vi "rad_Deploy Application Image.vi"(7 "App Image Temp Folder":path=path "C:/dev/Architectures/Reference Designs/Application Deployment and Replication/Application Deployment Utility/trunk/source/Application Images/_temp", 8 "error in (no error)":errorcluster, 10 "Selected Targets":T1[](array[typedef]) {"Primary NIC"."IP Address Request Mode" items=["Static"=1, "DHCP/Link-Local"=2, "Link-Local Only"=4, "DHCP Only"=8]}, 11 "App Image Path":path=path "C:/dev/Architectures/Reference Designs/Application Deployment and Replication/Application Deployment Utility/trunk/source/Application Images/AppImage1.lvappimg") -> (0 "error out":errorcluster, 1 "Cancelled":bool)   [LabVIEW 2020]
uses:
  TypeDefs/rad_Target Configuration Operations.ctl
  TypeDefs/rad_Deployment Status Data Type.ctl
  Util/FP Control/FP Control Functions.ctl
  TypeDefs/rad_Deployment Progress Data Type.ctl
  TypeDefs/rad_Deployment Notifiers.ctl
  <vilib>/nisyscfg/nisyscfg.lvlib
  <vilib>/nisyscfg/Close (System).vi
  support/SubVIs/Target Information.ctl
  Targets/TypeDefs/rad_Target Network Settings.ctl
  TypeDefs/rad_Target Configuration Settings.ctl
panel:
  in  "Configure Targets":bool
  out "Stop Updates":bool
  in  "Deploy":bool
  in  "Log":bool
  in  "Stop":bool
  in  "State Variables":T6={"App Image Path"=path "C:/dev/Architectures/Reference Designs/Application Deployment and Replication/Application Deployment Utility/trunk/source/Application Images/AppImage1.lvappimg", "App Image Temp Folder"=path "C:/dev/Architectures/Reference Designs/Application Deployment and Replication/Application Deployment Utility/trunk/source/Application Images/_temp", "Targets"=[], "Target Configuration Options"={"NumInBatch"=0, "Target Config Operation"=enum."No Config", "Target Name"="", "Increment Static IPs"=FALSE, "Change Target Name"=FALSE, "Primary NIC"={"MAC address"="", "IP Address Request Mode"=2, "IP address"="", "Subnet mask"="", "Gateway"="", "DNS server"=""}}, "Deployment Notifiers"=[]} {"Target Configuration Options"."Primary NIC"."IP Address Request Mode" items=["Static"=1, "DHCP/Link-Local"=2, "Link-Local Only"=4, "DHCP Only"=8]; "Targets"."Primary NIC"."IP Address Request Mode" items=["Static"=1, "DHCP/Link-Local"=2, "Link-Local Only"=4, "DHCP Only"=8]}
  out "Targets":i32(listbox)
  in  "Close":bool
  # "Targets"
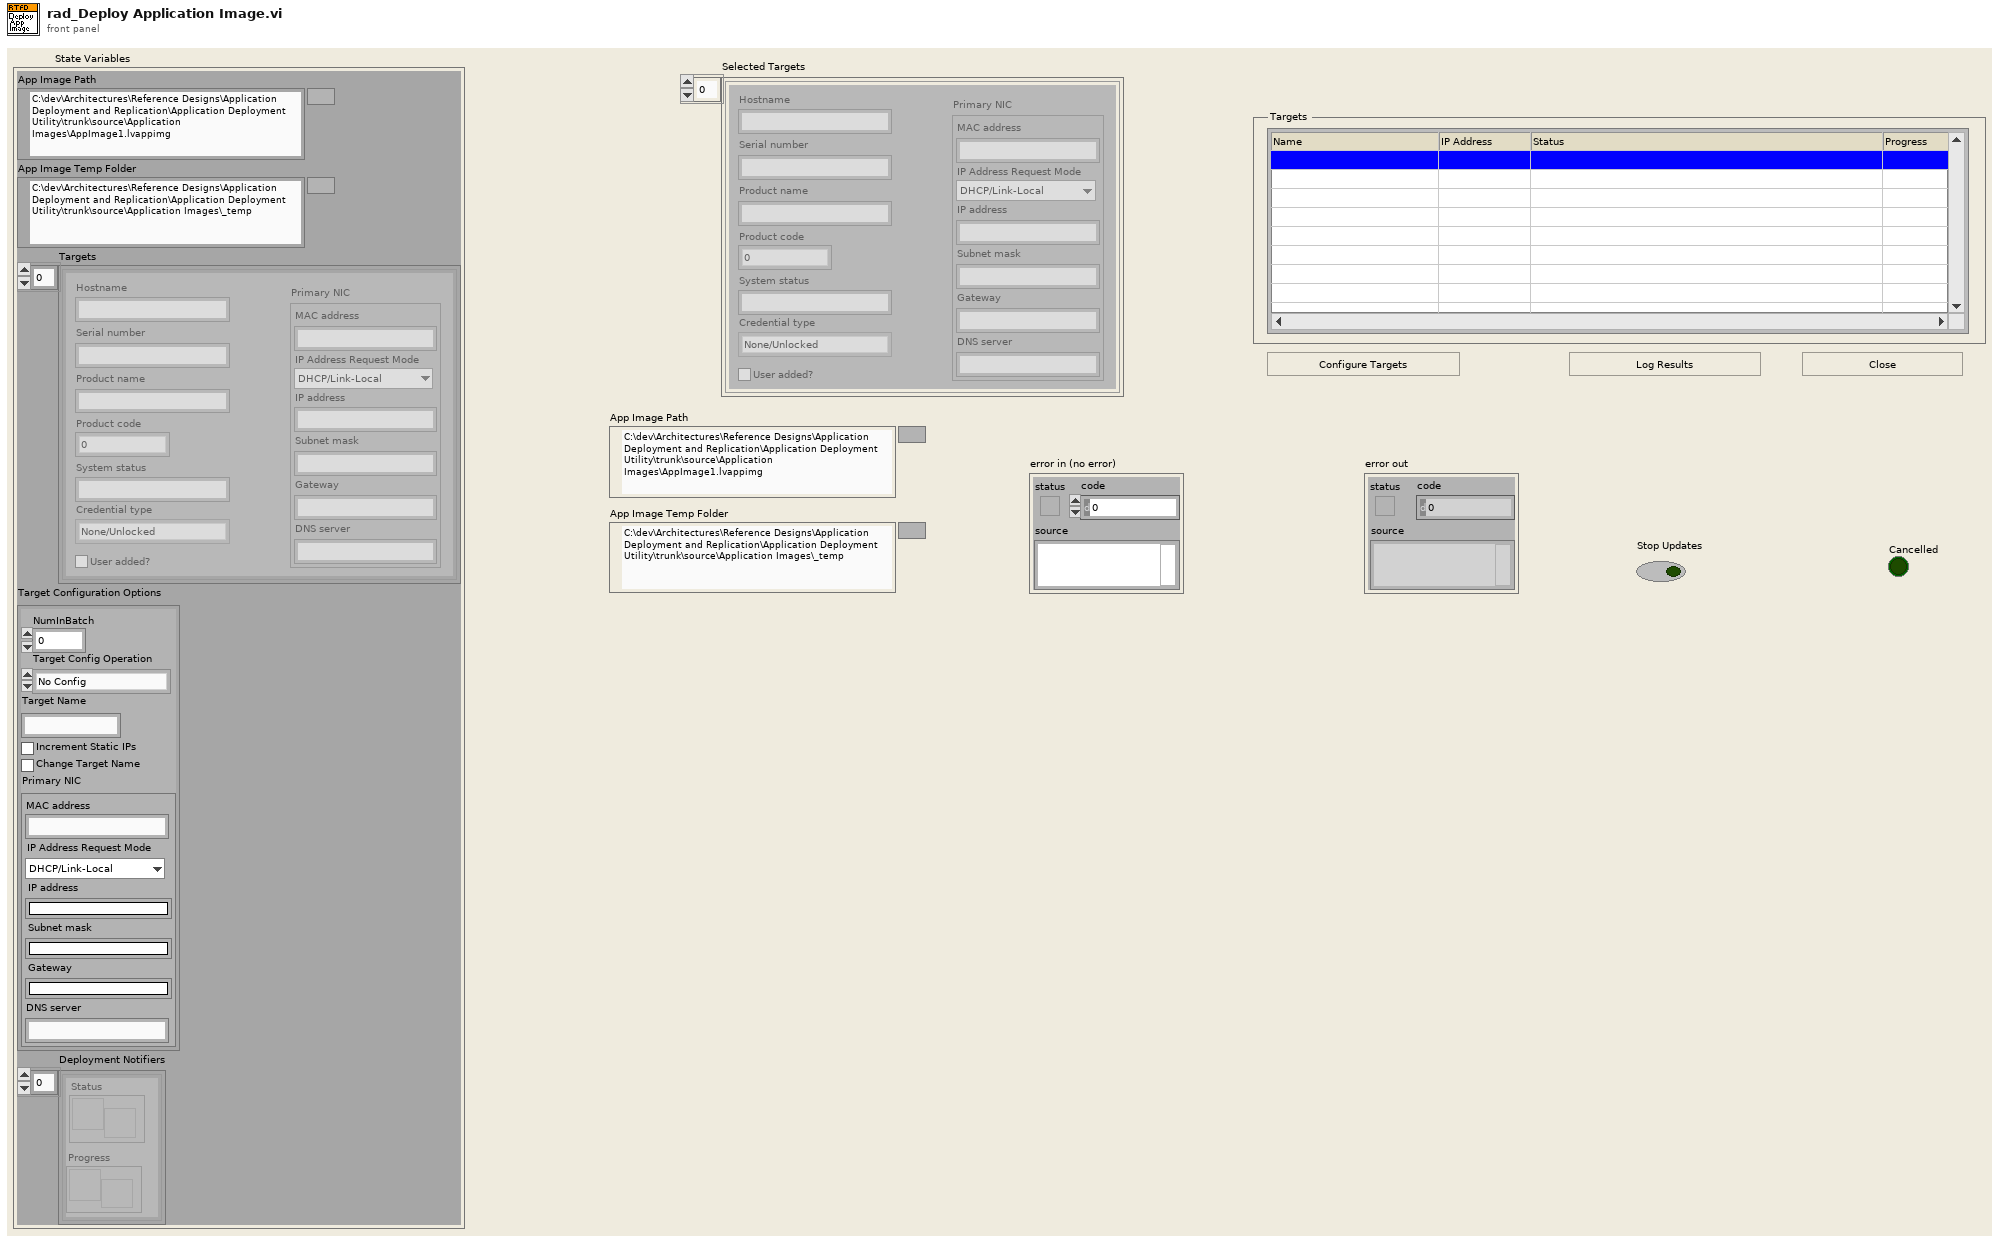
[diagram p1: front panel]
types:
  T1 = typedef "Target Information.ctl" = cluster{"Hostname":string, "Serial number":string, "Product name":string, "Product code":i32, "System status":string, "Credential type":enum16{"None/Unlocked", "FTP Password", "NIAuth Credentials"}, "User added?":bool, "Primary NIC":T2}
  T2 = typedef "rad_Target Network Settings.ctl" = cluster{"MAC address":string, "IP Address Request Mode":i32, "IP address":string, "Subnet mask":string, "Gateway":string, "DNS server":string}
  T3 = typedef "rad_Target Configuration Settings.ctl" = cluster{"NumInBatch":u32, "Target Config Operation":T4, "Target Name":string, "Increment Static IPs":bool, "Change Target Name":bool, "Primary NIC":T2}
  T4 = typedef "rad_Target Configuration Operations.ctl" = enum8{"No Config", "Image Config", "Static Config"}
  T5 = typedef "rad_Deployment Notifiers.ctl" = cluster{"Status":refnum<notifier>, "Progress":refnum<notifier>}
  T6 = cluster{"App Image Path":path, "App Image Temp Folder":path, "Targets":T1[], "Target Configuration Options":T3, "Deployment Notifiers":T5[]}
  T7 = typedef "rad_Deployment Progress Data Type.ctl" = i8
  T8 = typedef "rad_Deployment Status Data Type.ctl" = string
  T9 = typedef "FP Control Functions.ctl" = enum16{"Open", "Close", "Bring To Front", "Center"}
  T10 = enum8{"Enabled", "Disabled", "Disabled and Grayed Out"}
  T11 = typedef "rad_Application Image Properties.ctl" = cluster{"Name":string, "Version":string, "Time":timestamp, "Description":string, "Key":string, "Chassis":string, "FPGA Properties":T12, "Model":string, "Retrieve":string[], "Deploy":string[], "Installed Software":string[]}
  T12 = typedef "rad_FPGA Properties.ctl" = T13[]
  T13 = typedef "rad_FPGA Flash Properties.ctl" = cluster{"Resource Name":string, "Path":path}
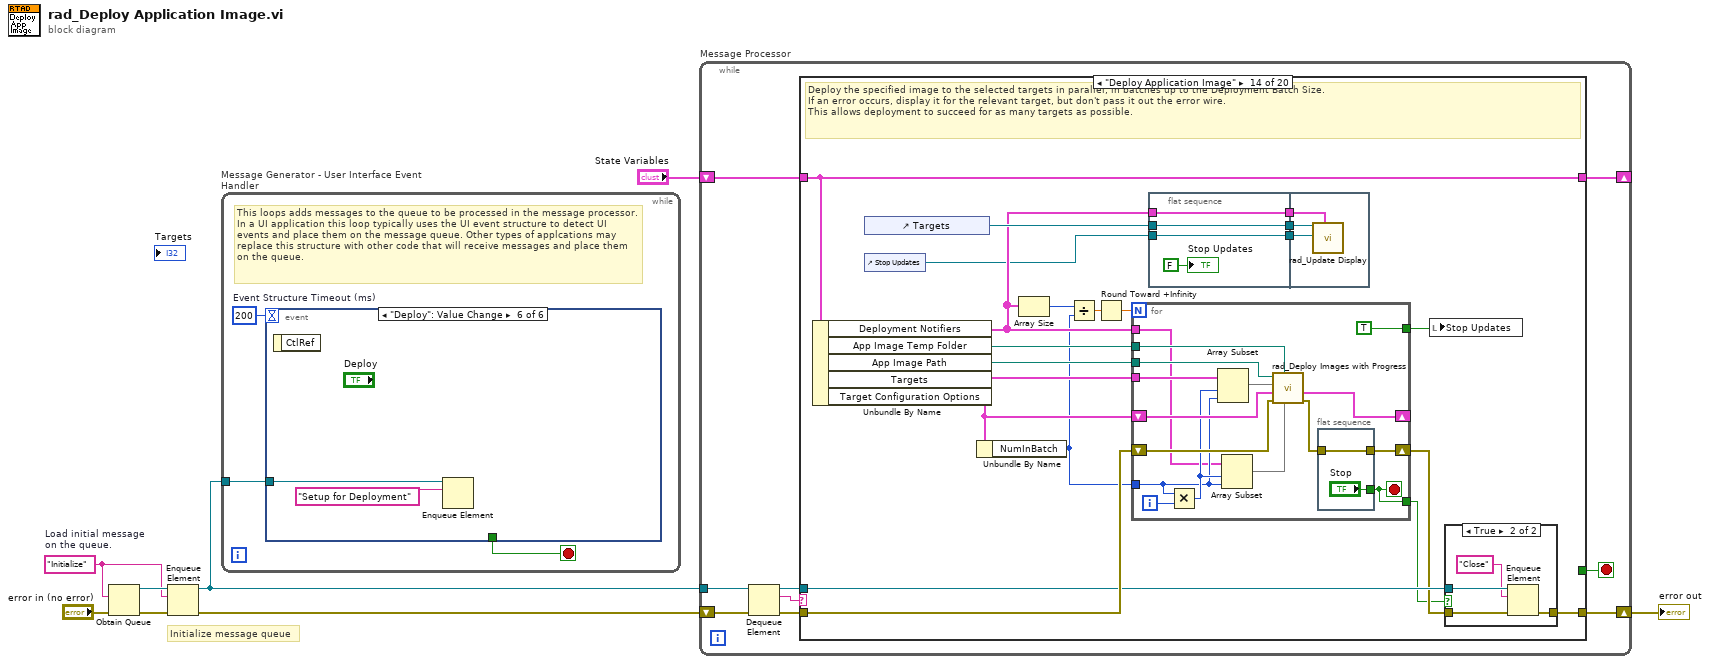
[diagram p0: block diagram]
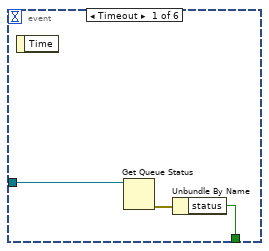
[diagram p2: hidden frame]
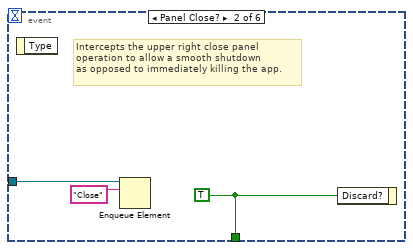
[diagram p3: hidden frame]
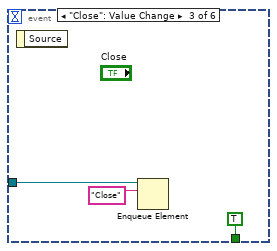
[diagram p4: hidden frame]
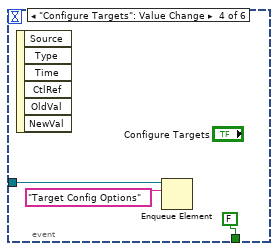
[diagram p5: hidden frame]
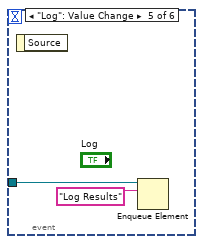
[diagram p6: hidden frame]
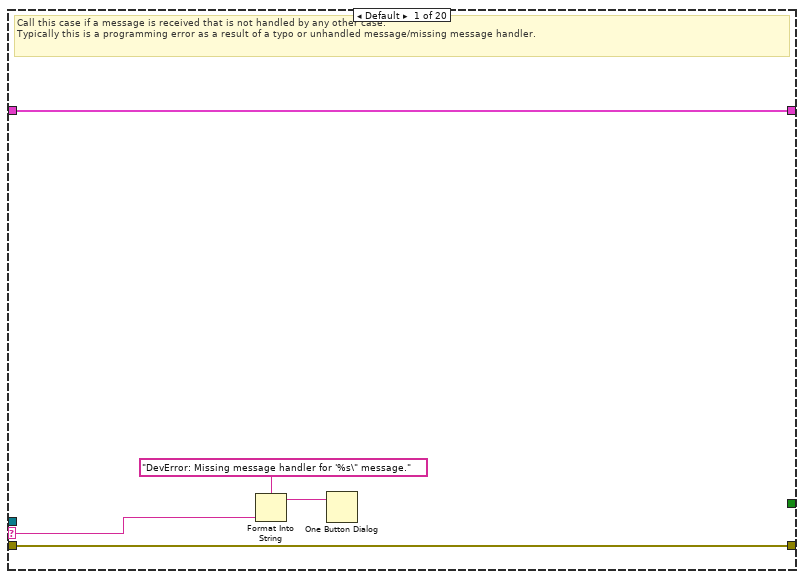
[diagram p7: hidden frame]
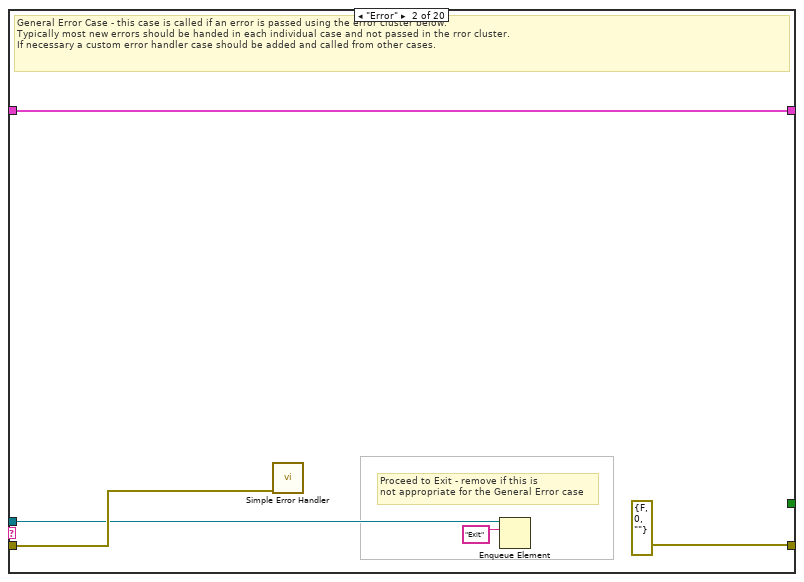
[diagram p8: hidden frame]
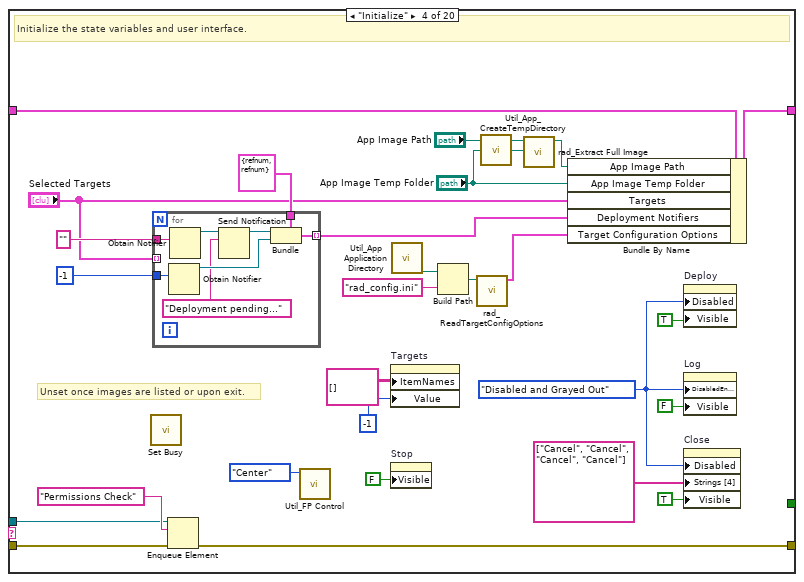
[diagram p10: hidden frame]
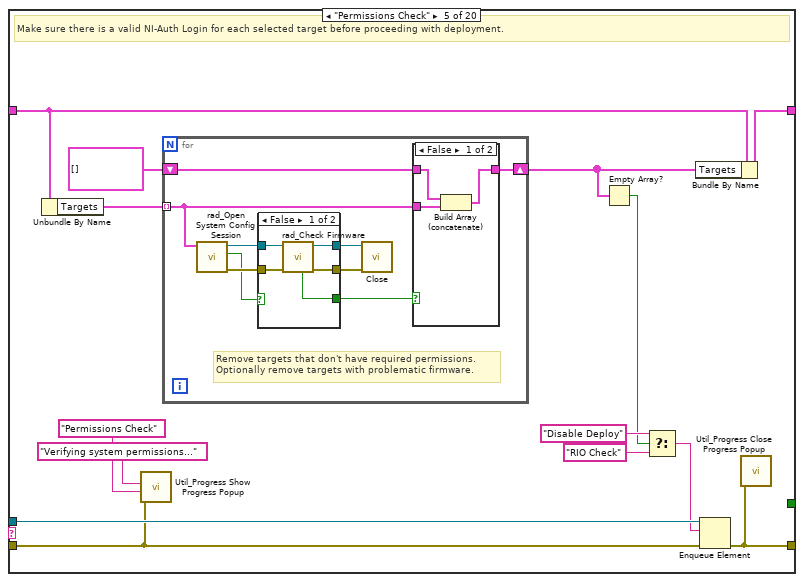
[diagram p11: hidden frame]
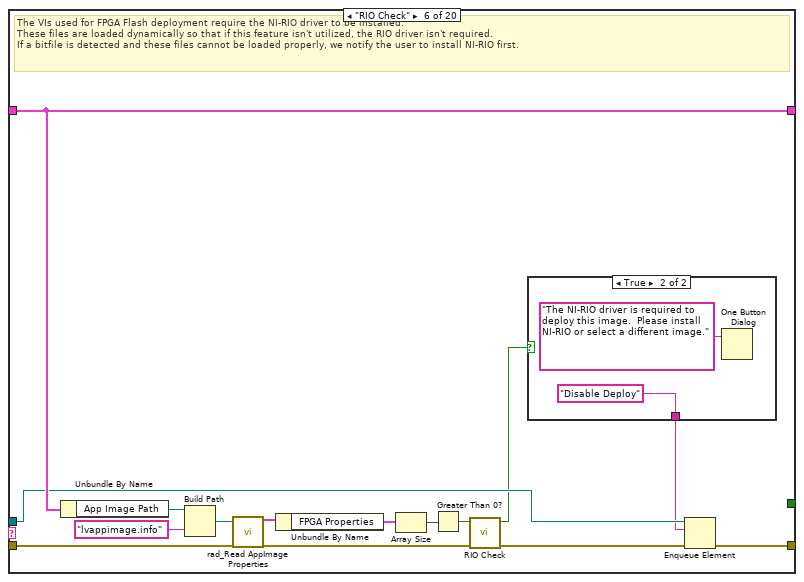
[diagram p14: hidden frame]
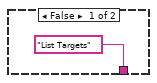
[diagram p15: hidden frame]
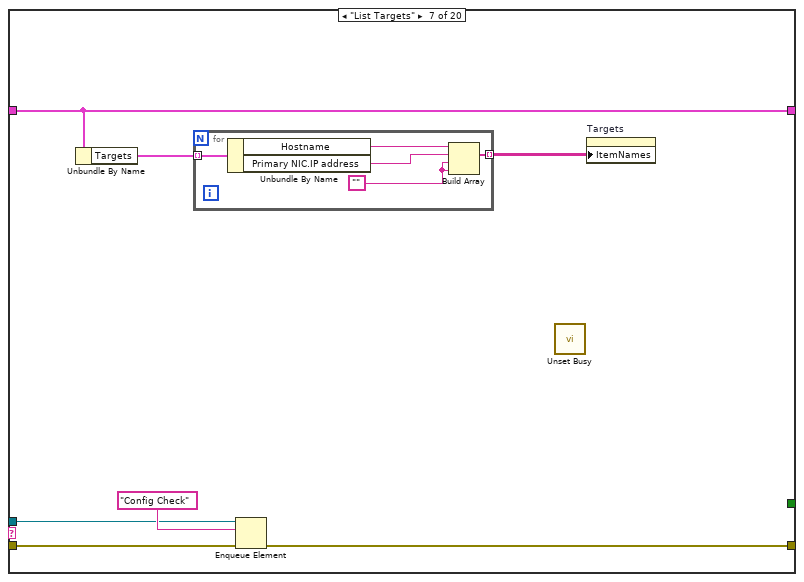
[diagram p16: hidden frame]
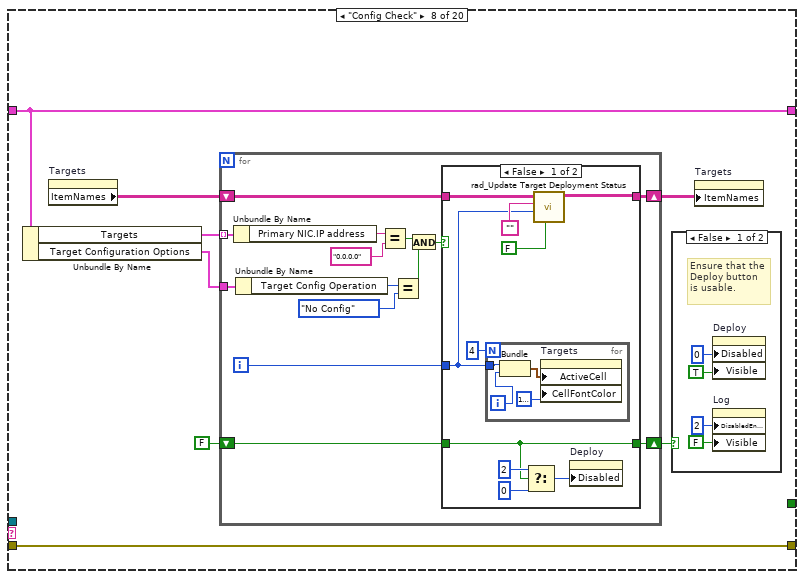
[diagram p17: hidden frame]
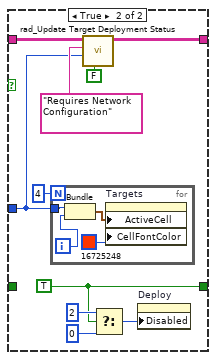
[diagram p19: hidden frame]
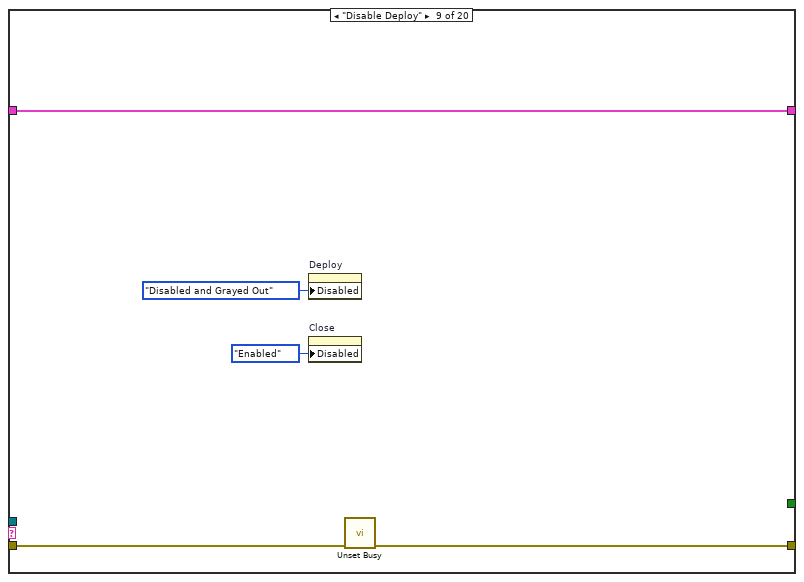
[diagram p20: hidden frame]
diagram:
  w1 = "Initialize"  # Load initial message on the queue.
  # "Initialize message queue"
  n1 = Obtain Queue(element data type=w1, error in (no error)="error in (no error)") -> (queue out=w3:refnum<queue>, error out=w8:errorcluster)  [unwired: 3 in, 1 out]
  n2 = Enqueue Element(queue=w3, element=w1, error in (no error)=w8) -> (queue out=w2:refnum<queue>, error out=w4:errorcluster)  [unwired: 1 in, 1 out]
  n3 = while "Message Generator - User Interface Event Handler" {
    tunnel: w2 -> [w9]
    stop <- w10 stop-if-true
    w11 = 200  # Event Structure Timeout (ms)
    # "This loops adds messages to the queue to be processed in the message processor. In a UI application this loop typically uses the UI event structure to detect UI events and place them on the message queue. Other types of applcations may replace this structure with other code that will receive messages and place them on the queue."
    n4 = event shown="[5] \"Deploy\": Value Change" {
      selector: _ -> [_ _ _ _ _ _]
      dyn-events: _ -> [_ _ _ _ _ _]
      timeout: w11 -> [_ _ _ _ _ _]
      tunnel: [w13 w17 TRUE ("Discard?") FALSE ("Discard?") _ _] -> w10
      tunnel: w9 -> [w12 w16 w20 w23 w25 w27]
      event Timeout {
        n5 = event-data() -> ()  [unwired: 2 out]
        n6 = Get Queue Status(queue=w12) -> (error out=w14:errorcluster)  [unwired: 2 in, 7 out]
        n7 = Unbundle By Name(w14) -> ("status"=w13:bool)
      }
      event Panel Close? {
        w17 = TRUE ("Discard?")
        # "Intercepts the upper right close panel\noperation to allow a smooth shutdown\nas opposed to immediately killing the app."
        n8 = event-data() -> ()  [unwired: 2 out]
        n9 = Enqueue Element(queue=w16, element="Close") -> ()  [unwired: 2 in, 3 out]
        n10 = event-data("Discard?"=w17) -> ()  [unwired: 1 in, 1 out]
      }
      event "Close": Value Change {
        n11 = event-data() -> ()  [unwired: 2 out]
        n12 = Enqueue Element(queue=w20, element="Close") -> ()  [unwired: 2 in, 3 out]
      }
      event "Configure Targets": Value Change {
        n13 = event-data() -> ()  [unwired: 7 out]
        n14 = Enqueue Element(queue=w23, element="Target Config Options") -> ()  [unwired: 2 in, 3 out]
      }
      event "Log": Value Change {
        n15 = event-data() -> ()  [unwired: 2 out]
        n16 = Enqueue Element(queue=w25, element="Log Results") -> ()  [unwired: 2 in, 3 out]
      }
      event "Deploy": Value Change {
        n17 = event-data() -> ()  [unwired: 2 out]
        n18 = Enqueue Element(queue=w27, element="Setup for Deployment") -> ()  [unwired: 2 in, 3 out]
      }
    }
  }
  n19 = while "Message Processor" {
    shift-left: w4 -> [w31]
    shift-right: [w32] -> w5
    tunnel: w2 -> [w30]
    shift-left: "State Variables" -> [w36]
    shift-right: [w35] -> _
    stop <- w28 stop-if-true
    n20 = Dequeue Element(queue=w30, error in (no error)=w31) -> (queue out=w34:refnum<queue>, element=w29:string, error out=w33:errorcluster)  [unwired: 1 in, 1 out]
    n21 = case shown="\"Deploy Application Image\"" w29 {
      selector: w29 -> [w39 _ _ _ _ _ _ _ _ _ _ _ _ _ _ _ _ _ _ _]
      tunnel: [w41 w46 w48 w75 w95 w131 w142 w152 w206 w210 w212 w218 w238 w257 w294 w302 w304 w312 w315 w322] -> w35
      tunnel: w36 -> [w41 w46 w48 w76 w96 w131 w142 w152 w206 w210 w212 w219 w238 w257 w294 w302 w304 w312 w315 w322]
      tunnel: w34 -> [_ w43 _ w54 w94 w128 w138 _ _ _ _ w216 w234 w252 _ _ _ w306 _ w327]
      tunnel: w33 -> [w40 w44 w47 w70 w90 w123 w140 w157 w208 w209 w211 w220 w239 w256 w295 w300 w303 w307 w313 w328]
      tunnel: [w40 errorcluster {"status"=FALSE, "code"=0, "source"=""} ("error out") w47 w56 w89 w129 w139 w157 w207 w209 w211 w214 w230 w250 w295 w299 w303 w305 w313 w319] -> w32
      tunnel: [_ _ _ _ _ _ _ _ _ _ _ _ _ _ _ _ _ _ _ TRUE] -> w28
      frame Default {
        # "Call this case if a message is received that is not handled by any other case.\nTypically this is a programming error as a result of a typo or unhandled message/missing message handler."
        n22 = Format Into String(format string="DevError: Missing message handler for '%s\" message." ("message"), w39) -> (resulting string=w37:string)  [unwired: 2 in, 1 out]
        n23 = One Button Dialog(message=w37) -> ()  [unwired: 2 out]
      }
      frame "Error" {
        # "Proceed to Exit - remove if this is\nnot appropriate for the General Error case"
        # "General Error Case - this case is called if an error is passed using the error cluster below.\nTypically most new errors should be handed in each individual case and not passed in the rror cluster.\nIf necessary a custom error handler case should be added and called from other cases."
        n24 = call <vilib>:"Simple Error Handler.vi"("error in (no error)"=w44) -> ()  [unwired: 1 in, 8 out]
        n25 = Enqueue Element(queue=w43, element="Exit") -> ()  [unwired: 2 in, 3 out]
      }
      frame "*******Init******" {
        # "Dummy case to add a seperator in the Case Structure menu."
      }
      frame "Initialize" {
        w49 = T10."Disabled and Grayed Out" ("Disabled")
        # "Unset once images are listed or upon exit."
        # "Initialize the state variables and user interface."
        n26 = call <vilib>:"Set Busy.vi"() -> ()  [unwired: 10 in, 2 out]
        n27 = for {
          tunnel: T8 "" ("status notifier data type") -> [w84]
          tunnel: T7 -1 ("Progress") -> [w83]
          tunnel: T5 {"Status"=refnum, "Progress"=refnum} ("Deployment Notifiers") -> [w81]
          tunnel: [w80] -> w65 mode=indexing
          tunnel: "Selected Targets" -> [_] mode=indexing
          n28 = Obtain Notifier(notification data type=w83) -> (notifier out=w82:refnum<notifier>)  [unwired: 3 in, 2 out]
          n29 = Obtain Notifier(notification data type=w84) -> (notifier out=w79:refnum<notifier>)  [unwired: 3 in, 2 out]
          n30 = Send Notification(notification=T8 "Deployment pending...", notifier=w79) -> (notifier out=w78:refnum<notifier>)  [unwired: 1 in, 1 out]
          n31 = Bundle(cluster=w81, "Status"=w78, "Progress"=w82) -> (w80:T5)
        }
        n32 = Enqueue Element(queue=w54, element="Permissions Check", error in (no error)=w70) -> (error out=w56:errorcluster)  [unwired: 1 in, 2 out]
        n33 = call "Util_FP Control.vi"("Function"=FP_Control_Functions."Center") -> ()  [unwired: 1 in, 10 out]
        n34 = property on="Targets" class="MCListbox (strict)"("ItemNames"=string[][] [] ("Item Names"), "Value"=-1 ("Targets")) -> ()  [unwired: 2 in, 2 out]
        n35 = property on="Stop" class="Bool"("Visible"=FALSE) -> ()  [unwired: 2 in, 2 out]
        n36 = call "Util_App Application Directory.vi"() -> ("Application Directory"=w64:path)  [unwired: 11 out]
        n37 = Build Path(base path=w64, name or relative path="rad_config.ini" ("Config File Name")) -> (appended path=w62:path)
        n38 = call "rad_ReadTargetConfigOptions.vi"("configuration file path"=w62) -> ("TargetConfigurationOptions"=w61:T3)  [unwired: 9 in, 1 out]
        n39 = call "Util_App_CreateTempDirectory.vi"("TempFolderPath"="App Image Temp Folder") -> ("TempFolderPath_out"=w58:path)
        n40 = call "rad_Extract Full Image.vi"("App Image Temp Folder"=w58, "Zipped App Image File Path"="App Image Path") -> ("Unzipped App Image Folder Path"=w59:path)  [unwired: 8 in, 1 out]
        n41 = Bundle By Name(cluster=w76, "App Image Path"=w59, "App Image Temp Folder"="App Image Temp Folder", "Targets"="Selected Targets", "Deployment Notifiers"=w65, "Target Configuration Options"=w61) -> (w75:T6)
        n42 = property on="Deploy" class="Bool"("Disabled"=w49, "Visible"=TRUE) -> ()  [unwired: 2 in, 2 out]
        n43 = property on="Log" class="Bool"("DisabledEnum"=w49, "Visible"=FALSE) -> ()  [unwired: 2 in, 2 out]
        n44 = property on="Close" class="Bool"("Disabled"=w49, "Strings [4]"=string[] ["Cancel", "Cancel", "Cancel", "Cancel"], "Visible"=TRUE) -> ()  [unwired: 2 in, 2 out]
      }
      frame "Permissions Check" {
        # "Make sure there is a valid NI-Auth Login for each selected target before proceeding with deployment."
        n45 = Unbundle By Name(w96) -> ("Targets"=w98:T1[])
        n46 = call "Util_Progress Show Progress Popup.vi"("error in (no error)"=w90, "Title"="Permissions Check" ("Message"), "Message"="Verifying system permissions...") -> ()  [unwired: 8 in, 1 out]
        n47 = for {
          tunnel: w98 -> [w105] mode=indexing
          shift-right: [w107] -> w86
          shift-left: T1[] [] -> [w106]
          # "Remove targets that don't have required permissions.\nOptionally remove targets with problematic firmware."
          n48 = call "rad_Open System Config Session.vi"("Target settings"=w105) -> ("error out"=w104:errorcluster, "Cancelled"=w99:bool, "Session out"=w102:refnum<k21>)  [unwired: 7 in, 1 out]
          n49 = case shown="False" w99 {
            selector: w99 -> [_ w113]
            tunnel: w104 -> [w112 w115]
            tunnel: [w109 w115] -> w103
            tunnel: w102 -> [w111 w114]
            tunnel: [w110 w114] -> w101
            tunnel: [w108 w113] -> w100
            frame False {
              n50 = call "rad_Check Firmware.vi"("error in (no error)"=w112, "System Configuration"=w111) -> ("error out"=w109:errorcluster, "System Configuration out"=w110:refnum<k21>, "Bad firmware and user canceled"=w108:bool)  [unwired: 7 in]
            }
            frame True {
            }
          }
          n51 = call-poly <vilib>:"Close.vi"("error in (no error)"=w103, "Session in"=w101) -> ()  [unwired: 9 in, 1 out]
          n52 = case shown="False" w100 {
            tunnel: w105 -> [w118 _]
            tunnel: [w117 w119] -> w107
            tunnel: w106 -> [w116 w119]
            frame False {
              n53 = Build Array (concatenate)(w116, w118) -> (w117:T1[])
            }
            frame True {
            }
          }
        }
        n54 = Empty Array?(array=w86) -> (empty?=w85:bool)
        n55 = Select(t="Disable Deploy", s=w85, f="RIO Check") -> (s? t:f=w91:string)
        n56 = Bundle By Name(cluster=w96, "Targets"=w86) -> (w95:T6)
        n57 = Enqueue Element(queue=w94, element=w91, error in (no error)=w90) -> (error out=w89:errorcluster)  [unwired: 1 in, 2 out]
        n58 = call "Util_Progress Close Progress Popup.vi"("error in (no error)"=w89) -> ()  [unwired: 10 in, 1 out]
      }
      frame "RIO Check" {
        # "The VIs used for FPGA Flash deployment require the NI-RIO driver to be installed.  \nThese files are loaded dynamically so that if this feature isn't utilized, the RIO driver isn't required.\nIf a bitfile is detected and these files cannot be loaded properly, we notify the user to install NI-RIO first."
        n59 = Unbundle By Name(w131) -> ("App Image Path"=w121:path)
        n60 = Build Path(base path=w121, name or relative path="lvappimage.info") -> (appended path=w120:path)
        n61 = call "rad_Read AppImage Properties.vi"("AppImage Properties Path"=w120, "error in (no error)"=w123) -> ("AppImage Properties"=w124:T11, "error out"=w125:errorcluster)  [unwired: 12 in, 4 out]
        n62 = Unbundle By Name(w124) -> ("FPGA Properties"=w134:T12)
        n63 = Array Size(array=w134) -> (size(s)=w133:i32)
        n64 = Greater Than 0?(x=w133) -> (x > 0?=w132:bool)
        n65 = call "RIO Check.vi"("error in"=w125, "Requires RIO"=w132) -> ("error out"=w130:errorcluster, "RIO needed but not installed"=w127:bool)  [unwired: 8 in]
        n66 = case shown="True" w127 {
          tunnel: ["List Targets" "Disable Deploy" ("t")] -> w126
          frame False {
          }
          frame True {
            n67 = One Button Dialog(message="The NI-RIO driver is required to deploy this image.  Please install NI-RIO or select a different image.") -> ()  [unwired: 1 in, 1 out]
          }
        }
        n68 = Enqueue Element(queue=w128, element=w126, error in (no error)=w130) -> (error out=w129:errorcluster)  [unwired: 1 in, 2 out]
      }
      frame "List Targets" {
        n69 = Unbundle By Name(w142) -> ("Targets"=w144:T1[])
        n70 = for {
          tunnel: w144 -> [w149] mode=indexing
          tunnel: [w146] -> w143 mode=indexing
          w145 = ""
          n71 = Unbundle By Name(w149) -> ("Hostname"=w148:string, "Primary NIC.IP address"=w147:string)
          n72 = Build Array(w148, w147, w145, w145) -> (w146:string[])
        }
        n73 = Enqueue Element(queue=w138, element="Config Check", error in (no error)=w140) -> (error out=w139:errorcluster)  [unwired: 1 in, 2 out]
        n74 = call <vilib>:"Unset Busy.vi"() -> ()  [unwired: 11 in, 1 out]
        n75 = property on="Targets" class="MCListbox (strict)"("ItemNames"=w143) -> ()  [unwired: 2 in, 2 out]
      }
      frame "Config Check" {
        n76 = Unbundle By Name(w152) -> ("Targets"=w155:T1[], "Target Configuration Options"=w156:T3)
        n77 = property on="Targets" class="MCListbox (strict)"() -> ("ItemNames"=w151:string[][])  [unwired: 2 in, 2 out]
        n78 = for {
          tunnel: w155 -> [w166] mode=indexing
          tunnel: w156 -> [w165]
          shift-right: [w162] -> w150
          shift-left: FALSE -> [w163]
          shift-right: [w168] -> w153
          shift-left: w151 -> [w164]
          i -> [w167]
          n79 = Unbundle By Name(w166) -> ("Primary NIC.IP address"=w175:string)
          n80 = Unbundle By Name(w165) -> ("Target Config Operation"=w173:T4)
          n81 = Equal?(x=w175, y="0.0.0.0") -> (x = y?=w171:bool)
          n82 = Equal?(x=w173, y=rad_Target_Configuration_Operations."No Config") -> (x = y?=w169:bool)
          n83 = And(x=w171, y=w169) -> (x .and. y?=w170:bool)
          n84 = case shown="False" w170 {
            tunnel: [w184 w199] -> w168
            tunnel: w167 -> [w182 w195]
            tunnel: w164 -> [w185 w196]
            tunnel: w163 -> [w177 _]
            tunnel: [w177 w192] -> w162
            frame False {
              n85 = for {
                N: 4 -> [_]
                tunnel: w182 -> [w188]
                i -> [w187]
                n86 = Bundle(w188, w187) -> (w186:cluster{i32, i32})  [unwired: 1 in]
                n87 = property on="Targets" class="MCListbox (strict)"("ActiveCell"=w186, "CellFontColor"=u32 16777222) -> ()  [unwired: 2 in, 2 out]
              }
              n88 = Select(t=2, s=w177, f=0) -> (s? t:f=w178:i32)
              n89 = call "rad_Update Target Deployment Status.vi"("Add Timestamp?"=FALSE, "Target Index"=w182, "Message"="", "Targets Deployment Status"=w185) -> ("Targets Deployment Status"=w184:string[][])  [unwired: 7 in]
              n90 = property on="Deploy" class="Bool"("Disabled"=w178) -> ()  [unwired: 2 in, 2 out]
            }
            frame True {
              w192 = TRUE
              n91 = for {
                N: 4 -> [_]
                tunnel: w195 -> [w202]
                i -> [w201]
                n92 = Bundle(w202, w201) -> (w200:cluster{i32, i32})  [unwired: 1 in]
                n93 = property on="Targets" class="MCListbox (strict)"("ActiveCell"=w200, "CellFontColor"=u32 16725248) -> ()  [unwired: 2 in, 2 out]
              }
              n94 = call "rad_Update Target Deployment Status.vi"("Add Timestamp?"=FALSE, "Target Index"=w195, "Message"="Requires Network Configuration", "Targets Deployment Status"=w196) -> ("Targets Deployment Status"=w199:string[][])  [unwired: 7 in]
              n95 = Select(t=2, s=w192, f=0) -> (s? t:f=w191:i32)
              n96 = property on="Deploy" class="Bool"("Disabled"=w191) -> ()  [unwired: 2 in, 2 out]
            }
          }
        }
        n97 = case shown="False" w150 {
          frame False {
            # "Ensure that the\nDeploy button\nis usable."
            n98 = property on="Deploy" class="Bool"("Disabled"=0, "Visible"=TRUE) -> ()  [unwired: 2 in, 2 out]
            n99 = property on="Log" class="Bool"("DisabledEnum"=2, "Visible"=FALSE) -> ()  [unwired: 2 in, 2 out]
          }
          frame True {
          }
        }
        n100 = property on="Targets" class="MCListbox (strict)"("ItemNames"=w153) -> ()  [unwired: 2 in, 2 out]
      }
      frame "Disable Deploy" {
        n101 = property on="Deploy" class="Bool"("Disabled"=T10."Disabled and Grayed Out") -> ()  [unwired: 2 in, 2 out]
        n102 = property on="Close" class="Bool"("Disabled"=T10."Enabled") -> ()  [unwired: 2 in, 2 out]
        n103 = call <vilib>:"Unset Busy.vi"("error in (no error)"=w208) -> ("error out"=w207:errorcluster)  [unwired: 10 in]
      }
      frame "*****************" {
        # "Dummy case to add a seperator in the Case Structure menu."
      }
      frame "Update Display" {
      }
      frame "Target Config Options" {
        # "Update the options for the network configuration settings which may be applied to each RT target after deploying the application image."
        n104 = Unbundle By Name(w219) -> ("Target Configuration Options"=w221:T3)
        n105 = call "rad_Target Configuration Options Dialog.vi"("error in"=w220, "Target Configuration Options"=w221) -> ("error out"=w215:errorcluster, "Cancelled"=w213:bool, "Target Configuration Options"=w217:T3)  [unwired: 7 in]
        n106 = case shown="False" w213 {
          tunnel: w216 -> [w225 _]
          tunnel: w215 -> [w224 w226]
          tunnel: [w223 w226] -> w214
          frame False {
            n107 = Enqueue Element(queue=w225, element="Config Check" ("Message Name"), error in (no error)=w224) -> (error out=w223:errorcluster)  [unwired: 1 in, 2 out]
          }
          frame True {
          }
        }
        n108 = Bundle By Name(cluster=w219, "Target Configuration Options"=w217) -> (w218:T6)
      }
      frame "Setup for Deployment" {
        w236 = T10."Disabled and Grayed Out" ("Disabled")
        # "Update the UI for the deployment process - disable some buttons."
        n109 = Enqueue Element(queue=w234, element="Deploy Application Image", error in (no error)=w239) -> (queue out=w231:refnum<queue>, error out=w232:errorcluster)  [unwired: 1 in, 1 out]
        n110 = property on="Stop" class="Bool"("Visible"=TRUE) -> ()  [unwired: 2 in, 2 out]
        n111 = property on="Close" class="Bool"("Disabled"=w236, "Visible"=FALSE) -> ()  [unwired: 2 in, 2 out]
        n112 = property on="Log" class="Bool"("Disabled"=w236, "Visible"=TRUE) -> ()  [unwired: 2 in, 2 out]
        n113 = Enqueue Element(queue=w231, element="Cleanup from Deployment", error in (no error)=w232) -> (error out=w230:errorcluster)  [unwired: 1 in, 2 out]
        n114 = property on="Deploy" class="Bool"("Visible"=FALSE) -> ()  [unwired: 2 in, 2 out]
      }
      frame "Deploy Application Image" {
        # "Deploy the specified image to the selected targets in parallel, in batches up to the Deployment Batch Size.\nIf an error occurs, display it for the relevant target, but don't pass it out the error wire.\nThis allows deployment to succeed for as many targets as possible."
        n115 = Unbundle By Name(w257) -> ("Deployment Notifiers"=w247:T5[], "App Image Temp Folder"=w258:path, "App Image Path"=w260:path, "Targets"=w259:T1[], "Target Configuration Options"=w241:T3)
        n116 = control-ref of="Targets"() -> (w248:refnum<vi>)
        n117 = control-ref of="Stop Updates"() -> (w243:refnum<vi>)
        n118 = Unbundle By Name(w241) -> ("NumInBatch"=w240:u32)
        n119 = Array Size(array=w247) -> (size(s)=w255:i32)
        n120 = Divide(x=w255, y=w240) -> (x/y=w254:dbl)
        n121 = Round Toward +Infinity(x=w254) -> (ceil(x): smallest int >= x=w253:dbl)
        n122 = for {
          N: w253 -> [_]
          tunnel: w260 -> [w287]
          tunnel: w259 -> [w282]
          tunnel: w258 -> [w286]
          tunnel: w240 -> [w279]
          shift-right: [w278] -> w251
          shift-left: w256 -> [w285]
          tunnel: [w276] -> w249
          tunnel: w247 -> [w275]
          tunnel: [TRUE] -> w246
          shift-right: [w273] -> _
          shift-left: w241 -> [w288]
          i -> [w284]
          stop <- w276 stop-if-true
          n123 = Multiply(x=w279, y=w284) -> (x*y=w280:u32)
          n124 = Array Subset(array=w282, index=w280, length=w279) -> (w281:T1[])
          n125 = Array Subset(array=w275, index=w280, length=w279) -> (w283:T5[])
          n126 = call "rad_Deploy Images with Progress.vi"("Deployment Notifiers"=w283, "temp folder"=w286, "error in (no error)"=w285, "Target Config Options in"=w288, "RT Deployment Targets in"=w281, "image path"=w287) -> ("error out"=w277:errorcluster, "Target Config Options out"=w273:T3)  [unwired: 3 in, 1 out]
          n127 = flat-sequence {
            tunnel: ["Stop"] -> w276
            tunnel: [w289] -> w278
            tunnel: w277 -> [w289]
            frame #0 {
            }
          }
        }
        n128 = flat-sequence {
          tunnel: w247 -> [w263]
          tunnel: w248 -> [w264]
          tunnel: [w264] -> w245
          tunnel: [w263] -> w244
          tunnel: w243 -> [w262]
          tunnel: [w262] -> w242
          tunnel: w245 -> [w267]
          tunnel: w244 -> [w266]
          tunnel: w242 -> [w265]
          frame #0 {
            "Stop Updates" <- FALSE ("Stop Updates")
          }
          frame #1 {
            n129 = call "rad_Update Display.vi"("Deployment Notifiers"=w266, "Stop Updates"=w265, "Listbox Reference"=w267) -> ()  [unwired: 9 in]
          }
        }
        n130 = local write "Stop Updates"(w246) -> ()
        n131 = case shown="True" w249 {
          tunnel: w252 -> [_ w272]
          tunnel: w251 -> [w268 w271]
          tunnel: [w268 w270] -> w250
          frame False {
          }
          frame True {
            n132 = Enqueue Element(queue=w272, element="Close" ("Message Name"), error in (no error)=w271) -> (error out=w270:errorcluster)  [unwired: 1 in, 2 out]
          }
        }
      }
      frame "Cleanup from Deployment" {
        w292 = T10."Enabled" ("Disabled")
        # "Reset the UI after the deployment process."
        n133 = property on="Log" class="Bool"("Disabled"=w292) -> ()  [unwired: 2 in, 2 out]
        n134 = property on="Close" class="Bool"("Disabled"=w292, "Strings [4]"=string[] ["Close", "Close", "Close", "Close"], "Visible"=TRUE) -> ()  [unwired: 2 in, 2 out]
        n135 = property on="Stop" class="Bool"("Visible"=FALSE) -> ()  [unwired: 2 in, 2 out]
      }
      frame "Log Results" {
        # "Log the deployment information and results to a TSV file."
        n136 = Unbundle By Name(w302) -> ("Targets"=w301:T1[], "App Image Path"=w298:path)
        n137 = property on="Targets" class="MCListbox (strict)"() -> ("ItemNames"=w297:string[][])  [unwired: 2 in, 2 out]
        n138 = call "rad_Write Deployment Results to File.vi"("error in"=w300, "App Image Path"=w298, "Targets Deployment"=w297, "Targets"=w301) -> ("error out"=w299:errorcluster)  [unwired: 1 in, 6 out]
      }
      frame "******Close******" {
        # "Dummy case to add a seperator in the Case Structure menu."
      }
      frame "Close" {
        n139 = Enqueue Element(queue=w306, element="Cleanup Temp App Image", error in (no error)=w307) -> (queue out=w309:refnum<queue>, error out=w310:errorcluster)  [unwired: 1 in, 1 out]
        n140 = Enqueue Element(queue=w309, element="Exit", error in (no error)=w310) -> (error out=w305:errorcluster)  [unwired: 1 in, 2 out]
      }
      frame "Cleanup Temp App Image" {
        # "Empty the temp folder used during deployment."
        n141 = Unbundle By Name(w315) -> ("App Image Temp Folder"=w314:path)
        n142 = Delete(path (use dialog)=w314, entire hierarchy (F)=TRUE) -> ()  [unwired: 1 in, 5 out]
      }
      frame "Exit" {
        n143 = Unbundle By Name(w322) -> ("Deployment Notifiers"=w321:T5[])
        n144 = Release Queue(queue=w327, force destroy? (F)=TRUE, error in (no error)=w328) -> (error out=w320:errorcluster)  [unwired: 2 out]
        n145 = for {
          tunnel: w321 -> [w334] mode=indexing
          shift-right: [w329] -> w319
          shift-left: w320 -> [w332]
          n146 = Unbundle By Name(w334) -> ("Status"=w333:refnum<notifier>, "Progress"=w331:refnum<notifier>)
          n147 = Release Notifier(notifier=w333, force destroy? (F)=TRUE, error in (no error)=w332) -> (error out=w330:errorcluster)  [unwired: 2 out]
          n148 = Release Notifier(notifier=w331, force destroy? (F)=TRUE, error in (no error)=w330) -> (error out=w329:errorcluster)  [unwired: 2 out]
        }
        n149 = property on="Close" class="Bool"() -> ("Strings [4]"=w326:string[])  [unwired: 2 in, 2 out]
        n150 = Index Array(array=w326) -> (element=w325:string)  [unwired: 1 in]
        n151 = Equal?(x="Cancel", y=w325) -> (x = y?=→"Cancelled":bool)
        n152 = call <vilib>:"Unset Busy.vi"() -> ()  [unwired: 11 in, 1 out]
      }
    }
  }
  "error out" <- w5
